vi "CANMessageHandler.vi"(6 "IDs":sgl[](array[numeric]), 7 "Action":enum16{"Init", "Write", "Read", "Close"}(ring), 8 "error in (no error)":errorcluster, 10 "CAN Frame":T1 {"type" items=["CAN Data", "CAN Remote"]; "identifier" format="%.0x"}) -> (0 "error out":errorcluster, 2 "CAN Frame":T1 {"type" items=["CAN Data", "CAN Remote"]; "identifier" format="%.0x"}, 4 "IDs":sgl[](array[numeric]))   [LabVIEW 2016, in "DSI-RT.lvlib"]
uses:
  DSI-RT.lvlib
  <vilib>/RioEmbeddedCAN/RioEmbeddedCAN.llb/CANFrameControl.ctl
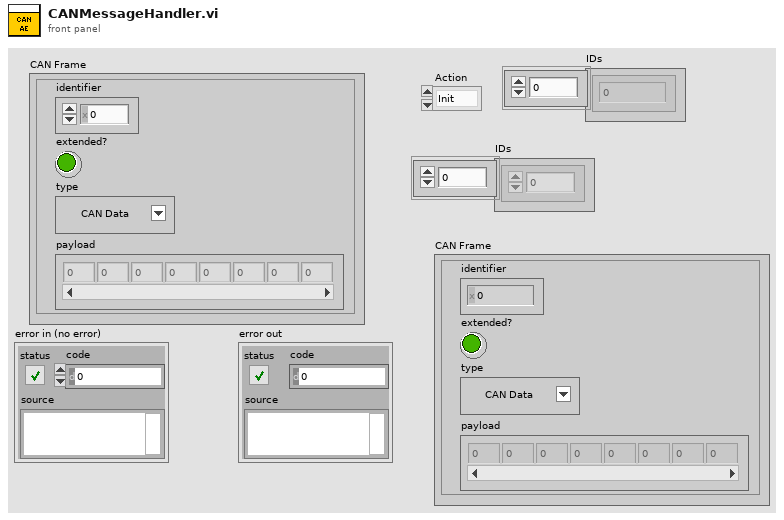
[diagram p1: front panel]
types:
  T1 = typedef "CANFrameControl.ctl" = cluster{"identifier":u32, "extended?":bool, "type":u8, "payload":u8[]}
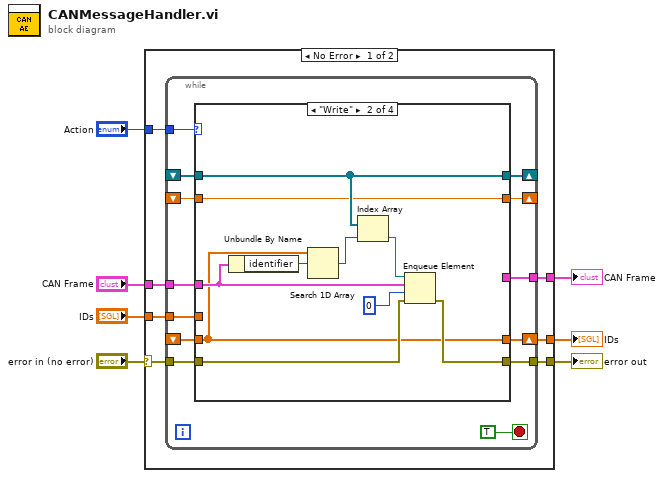
[diagram p0: block diagram]
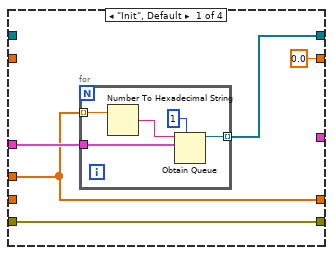
[diagram p2: hidden frame]
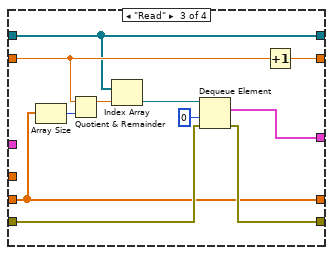
[diagram p3: hidden frame]
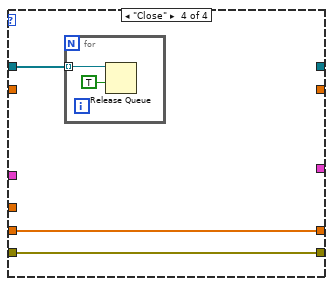
[diagram p4: hidden frame]
diagram:
  n1 = case shown="No Error" "error in (no error)" {
    selector: "error in (no error)" -> [w12 w65]
    tunnel: "Action" -> [w14 _]
    tunnel: "CAN Frame" -> [w13 _]
    tunnel: [w11 w65] -> w4
    tunnel: [w10 _] -> w3
    tunnel: "IDs" -> [w9 w64]
    tunnel: [w8 w64] -> w1
    frame No Error {
      n2 = while {
        tunnel: w14 -> [w27]
        shift-right: [w24] -> _
        shift-left: _ -> [w23]
        tunnel: w13 -> [w25]
        tunnel: w12 -> [w22]
        tunnel: [w21] -> w11
        tunnel: [w20] -> w10
        tunnel: w9 -> [w19]
        shift-right: [w18] -> _
        shift-left: _ -> [w17]
        shift-right: [w16] -> w8
        shift-left: _ -> [w15]
        stop <- TRUE stop-if-true
        n3 = case shown="\"Write\"" w27 {
          tunnel: w25 -> [w32 w42 _ _]
          tunnel: [w31 w46 w48 _] -> w24
          tunnel: w23 -> [_ w46 w48 w61]
          tunnel: w22 -> [w30 w40 w51 w60]
          tunnel: [w30 w39 w50 w60] -> w21
          tunnel: [_ _ w52 _] -> w20
          tunnel: w19 -> [w28 _ _ _]
          tunnel: [0.0 w41 w58 _] -> w18
          tunnel: w17 -> [_ w41 w57 _]
          tunnel: [w28 w38 w49 w59] -> w16
          tunnel: w15 -> [_ w38 w49 w59]
          frame "Init", Default {
            n4 = for {
              tunnel: w32 -> [w35]
              tunnel: [w34] -> w31 mode=indexing
              tunnel: w28 -> [w33] mode=indexing
              n5 = Number To Hexadecimal String(2:w33) -> (0:w36:string)  [unwired: 1 in]
              n6 = Obtain Queue(max queue size (-1, unlimited)=1, name (unnamed)=w36, element data type=w35) -> (queue out=w34:refnum<queue>)  [unwired: 2 in, 2 out]
            }
          }
          frame "Write" {
            n7 = Unbundle By Name(w42) -> ("identifier"=w45:u32)
            n8 = Search 1D Array(1D array=w38, element=w45) -> (index of element=w44:i32)  [unwired: 1 in]
            n9 = Index Array(array=w46, index=w44) -> (element=w43:refnum<queue>)
            n10 = Enqueue Element(queue=w43, element=w42, timeout in ms (-1)=0, error in (no error)=w40) -> (error out=w39:errorcluster)  [unwired: 2 out]
          }
          frame "Read" {
            n11 = Array Size(array=w49) -> (size(s)=w56:i32)
            n12 = Quotient & Remainder(x=w57, y=w56) -> (x-y*floor(x/y)=w55:dbl)  [unwired: 1 out]
            n13 = Index Array(array=w48, index=w55) -> (element=w54:refnum<queue>)
            n14 = Dequeue Element(queue=w54, timeout in ms (-1)=0, error in (no error)=w51) -> (element=w52:T1, error out=w50:errorcluster)  [unwired: 2 out]
            n15 = Increment(x=w57) -> (x+1=w58:dbl)
          }
          frame "Close" {
            n16 = for {
              tunnel: w61 -> [w63] mode=indexing
              n17 = Release Queue(queue=w63, force destroy? (F)=TRUE) -> ()  [unwired: 1 in, 3 out]
            }
          }
        }
      }
    }
    frame Error {
    }
  }
  "error out" <- w4
  "CAN Frame" <- w3
  "IDs" <- w1
